vi "ImageSize.vi"(8 "Error in":errorcluster caption="Error in (no error)", 11 "filename":path) -> (0 "Error out":errorcluster, 1 "imageHeight":i32, 2 "imageWidth":i32, 3 "filename out":path, 4 "landscape":bool)   [LabVIEW 2016]
panel:
  in  "uint32":u32
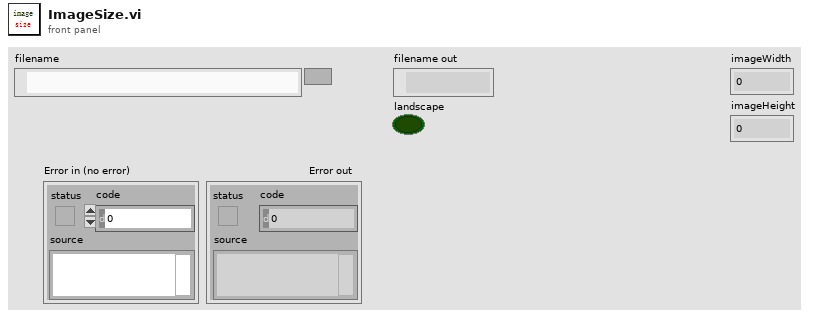
[diagram p1: front panel]
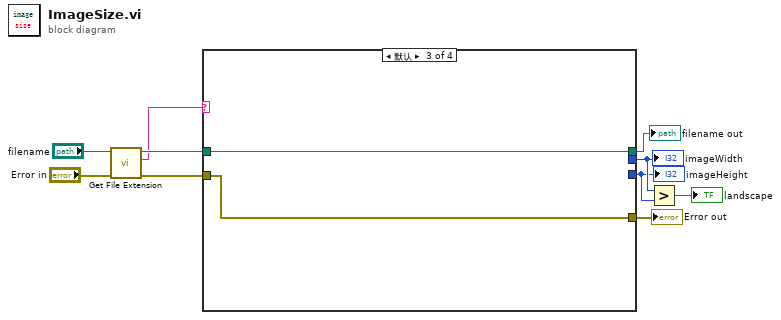
[diagram p0: block diagram]
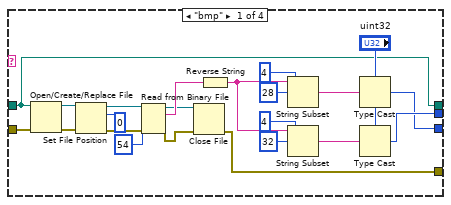
[diagram p2: hidden frame]
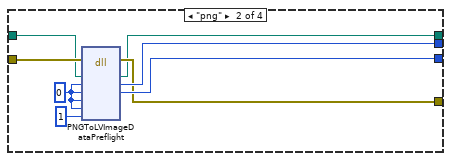
[diagram p3: hidden frame]
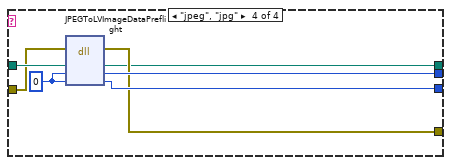
[diagram p4: hidden frame]
diagram:
  n1 = call <vilib>:"Get File Extension.vi"("error in (no error)"="Error in", "file"="filename") -> ("error out"=w6:errorcluster, "lowercase file extension"=w8:string, "dup file"=w9:path)  [unwired: 5 in, 2 out]
  n2 = case shown="默认" w8 {
    tunnel: w9 -> [w11 w37 w41 w48]
    tunnel: [w15 w36 _ w47] -> w3
    tunnel: [w14 w35 _ w46] -> w2
    tunnel: w6 -> [w13 w38 w42 w45]
    tunnel: [w12 w34 w42 w44] -> w5
    tunnel: [w11 w33 w41 w43] -> w4
    frame "bmp" {
      n3 = Open/Create/Replace File(file path (use dialog)=w11, error in=w13) -> (refnum out=w32:refnum<file>, error out=w31:errorcluster)  [unwired: 4 in, 1 out]
      n4 = Set File Position(offset (in bytes) (0)=0, refnum=w32, error in=w31) -> (refnum out=w29:refnum<file>, error out=w30:errorcluster)  [unwired: 1 in]
      n5 = Read from Binary File(8:w30, 10:54, 11:w29) -> (0:w17:errorcluster, 2:w24:string, 3:w16:refnum<file>)  [unwired: 3 in, 1 out]
      n6 = Close File(refnum=w16, error in=w17) -> (error out=w12:errorcluster)  [unwired: 1 out]
      n7 = Reverse String(1:w24) -> (0:w26:string)
      n8 = String Subset(string=w26, offset (0)=28, length (rest)=4) -> (substring=w27:string)
      n9 = String Subset(string=w26, offset (0)=32, length (rest)=4) -> (substring=w28:string)
      n10 = Type Cast(type="uint32", x=w27) -> (*(type *) &x=w14:u32)
      n11 = Type Cast(type="uint32", x=w28) -> (*(type *) &x=w15:u32)
    }
    frame "png" {
      w39 = 0 ("imageWidth")
      n12 = dll-call lib="LabVIEW" fn="PNGToLVImageDataPreflight"(error in=w38, "path to PNG file"=w37, "imageWidth"=w39, "imageHeight"=w39, "depth"=w39, "rowBytes"=w39, "padForPicture"=1 ("imageWidth")) -> (error out=w34:errorcluster, "path to PNG file"=w33:path, "imageWidth"=w36:i32, "imageHeight"=w35:i32)  [unwired: 6 in, 1 out]
    }
    frame Default {
    }
    frame "jpeg", "jpg" {
      w49 = 0
      n13 = dll-call lib="LabVIEW" fn="JPEGToLVImageDataPreflight"(error in=w45, "filename"=w48, "imageWidth"=w49, "imageHeight"=w49) -> (error out=w44:errorcluster, "filename"=w43:path, "imageWidth"=w47:i32, "imageHeight"=w46:i32)  [unwired: 3 in, 1 out]
    }
  }
  "imageWidth" <- w3
  "imageHeight" <- w2
  "Error out" <- w5
  "filename out" <- w4
  n14 = Greater?(x=w3, y=w2) -> (0:→"landscape":bool)
